vi "LCOD_Stack Queue Component.vi"(5 "Command":T1, 6 "error in":errorcluster, 7 "Numeric In":i32, 8 "String In":string, 9 "GUI Command":T2) -> (0 "error out":errorcluster, 1 "Numeric Out":i32, 2 "String Out":string, 3 "GUI Command Out":T2, 4 "More Items?":bool)   [LabVIEW 2009]
doc: "DESCRIPTION\nGeneral purpose data VI, used for holding Results data on the current batch of tests.\n\nCOMMANDS\nNo Command : Default error condition displays dialog reporting location of error.\nInitialise Stack : Set up Array local with the contents of Array In and ProdTestResults with ProdTestResults In\nAdd To Top : Insert Results into Index 0\nAdd To Bottom : Append Results onto Index (Length)\nPop From Top : Index 0 to ProdTestResults Out, removing Index 0\nPop From Bottom : Index (Length - 1) to ProdTestResults Out removing Index (Length - 1)\nMore Items? : Output on More Items? boolean\nRead Top : Index 0 to ProdTestResults Out\nRead Bottom : Index (Length - 1) to ProdTestResults Out."
uses:
  LCOD_Stack Queue GUI Command.ctl
  LCOD_Queue Command.ctl
  LCOD_GUI Cluster.ctl
panel:
  # "Input"
  # "Output"
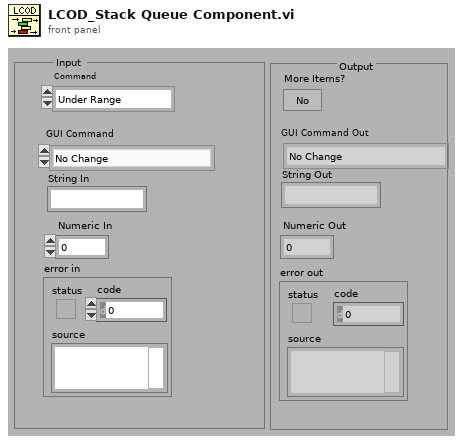
[diagram p1: front panel]
types:
  T1 = typedef "LCOD_Queue Command.ctl" = enum16{"Under Range", "Initialise Stack", "Add To Top", "Add To Bottom", "Pop From Bottom", "More Items?", "Read Bottom", "Over Range"}
  T2 = typedef "LCOD_Stack Queue GUI Command.ctl" = enum16{"No Change", "HadError", "ResetPressed", "DisplayMsg", "StartPressed", "SetGood", "SetNoGood", "SetIntesting"}
  T3 = typedef "LCOD_GUI Cluster.ctl" = cluster{"String":string, "Numeric":i32, "GUI Command":T2}
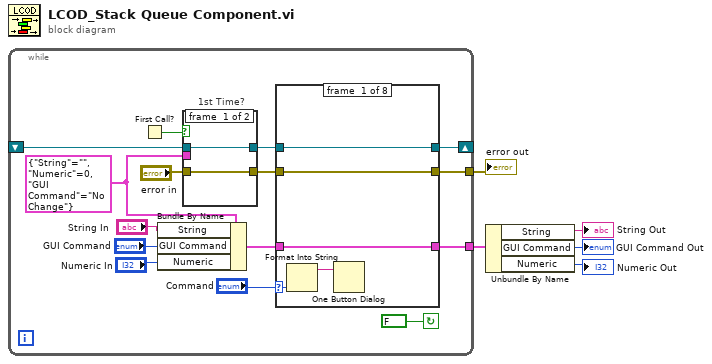
[diagram p0: block diagram]
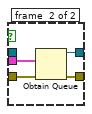
[diagram p2: hidden frame]
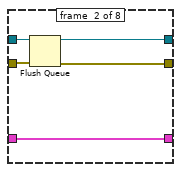
[diagram p3: hidden frame]
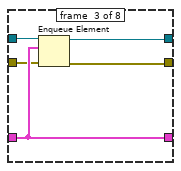
[diagram p4: hidden frame]
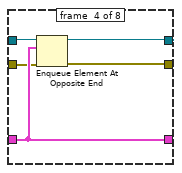
[diagram p5: hidden frame]
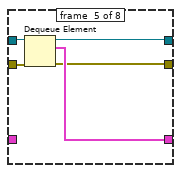
[diagram p6: hidden frame]
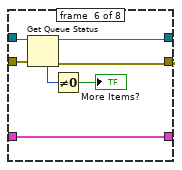
[diagram p7: hidden frame]
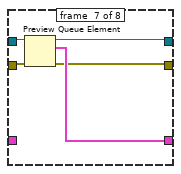
[diagram p8: hidden frame]
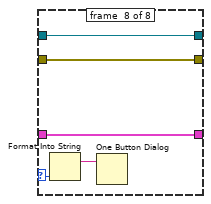
[diagram p9: hidden frame]
diagram:
  n1 = while {
    shift-right: [w16] -> _
    shift-left: _ -> [w15]
    tunnel: [w13] -> w5
    tunnel: [w11] -> w3
    stop <- FALSE continue-if-true
    w8 = T3 {"String"="", "Numeric"=0, "GUI Command"=enum."No Change"} ("ProdTestResults In")
    n2 = First Call?() -> (First Call?: T/F=w18:bool)
    n3 = Bundle By Name(cluster=w8, "String"="String In", "GUI Command"="GUI Command", "Numeric"="Numeric In") -> (w19:T3)
    n4 = case "1st Time?" shown="True" w18 {
      tunnel: w8 -> [_ w26]
      tunnel: [w22 w25] -> w17
      tunnel: w15 -> [w22 _]
      tunnel: [w21 w24] -> w12
      tunnel: "error in" -> [w21 w23]
      frame #0 {
      }
      frame #1 {
        n5 = Obtain Queue(element data type=w26, error in (no error)=w23) -> (queue out=w25:refnum<queue>, error out=w24:errorcluster)  [unwired: 2 in, 2 out]
      }
    }
    n6 = case shown="\"Over Range\"" "Command" {
      selector: "Command" -> [w31 _ _ _ _ _ _ w68]
      tunnel: w19 -> [w28 w34 w39 w44 _ w56 _ w65]
      tunnel: w17 -> [w29 w36 w41 w46 w51 w58 w63 w66]
      tunnel: [w29 w35 w40 w45 w50 w57 w62 w66] -> w16
      tunnel: [w28 w34 w39 w44 w49 w56 w61 w65] -> w13
      tunnel: w12 -> [w27 w33 w38 w43 w48 w54 w60 w64]
      tunnel: [w27 w32 w37 w42 w47 w53 w59 w64] -> w11
      frame #0 {
        n7 = Format Into String(w31) -> (resulting string=w30:string)  [unwired: 3 in, 1 out]
        n8 = One Button Dialog(message=w30) -> ()  [unwired: 2 out]
      }
      frame #1 {
        n9 = Flush Queue(queue=w36, error in (no error)=w33) -> (queue out=w35:refnum<queue>, error out=w32:errorcluster)  [unwired: 1 out]
      }
      frame #2 {
        n10 = Enqueue Element(queue=w41, element=w39, error in (no error)=w38) -> (queue out=w40:refnum<queue>, error out=w37:errorcluster)  [unwired: 2 out]
      }
      frame #3 {
        n11 = Enqueue Element At Opposite End(queue=w46, element=w44, error in (no error)=w43) -> (queue out=w45:refnum<queue>, error out=w42:errorcluster)  [unwired: 2 out]
      }
      frame #4 {
        n12 = Dequeue Element(queue=w51, error in (no error)=w48) -> (queue out=w50:refnum<queue>, element=w49:T3, error out=w47:errorcluster)  [unwired: 2 out]
      }
      frame #5 {
        n13 = Get Queue Status(queue=w58, error in (no error)=w54) -> (queue out=w57:refnum<queue>, error out=w53:errorcluster, # elements in queue=w55:i32)  [unwired: 6 out]
        n14 = Not Equal To 0?(x=w55) -> (x != 0?=→"More Items?":bool)
      }
      frame #6 {
        n15 = Preview Queue Element(queue=w63, error in (no error)=w60) -> (queue out=w62:refnum<queue>, element=w61:T3, error out=w59:errorcluster)  [unwired: 2 out]
      }
      frame #7 {
        n16 = Format Into String(w68) -> (resulting string=w67:string)  [unwired: 3 in, 1 out]
        n17 = One Button Dialog(message=w67) -> ()  [unwired: 2 out]
      }
    }
  }
  "error out" <- w3
  n18 = Unbundle By Name(w5) -> ("String"=→"String Out":string, "GUI Command"=→"GUI Command Out":T2, "Numeric"=→"Numeric Out":i32)
